vi "Hoff_cleaned.vi"(0 "Skip-1":i32=1, 2 "Image Pixels (U8)":u8[][](array[numeric])) -> (1 "3 times averaged":i32[][](graph), 5 "X Intercept":i32, 6 "Angle":i32, 7 "X Intercept 2":i32, 8 "Angle 2":i32)   [LabVIEW 2009]
panel:
  in  "Angle Canceling Resolution":i32=20
  in  "X Intercept Canceling Resolution":i32=200
  in  "Xintercept Pixel Resolution":dbl=20.0
  out "Vector Reformat":i32[][](array[numeric])
  out "Intensity Graph":i32[][](graph)
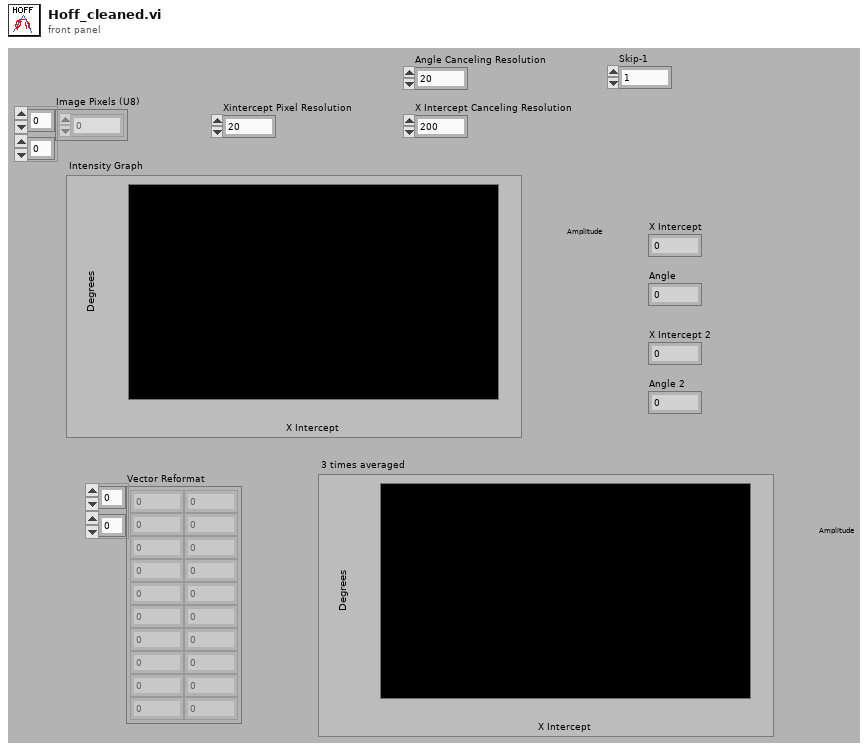
[diagram p1: front panel]
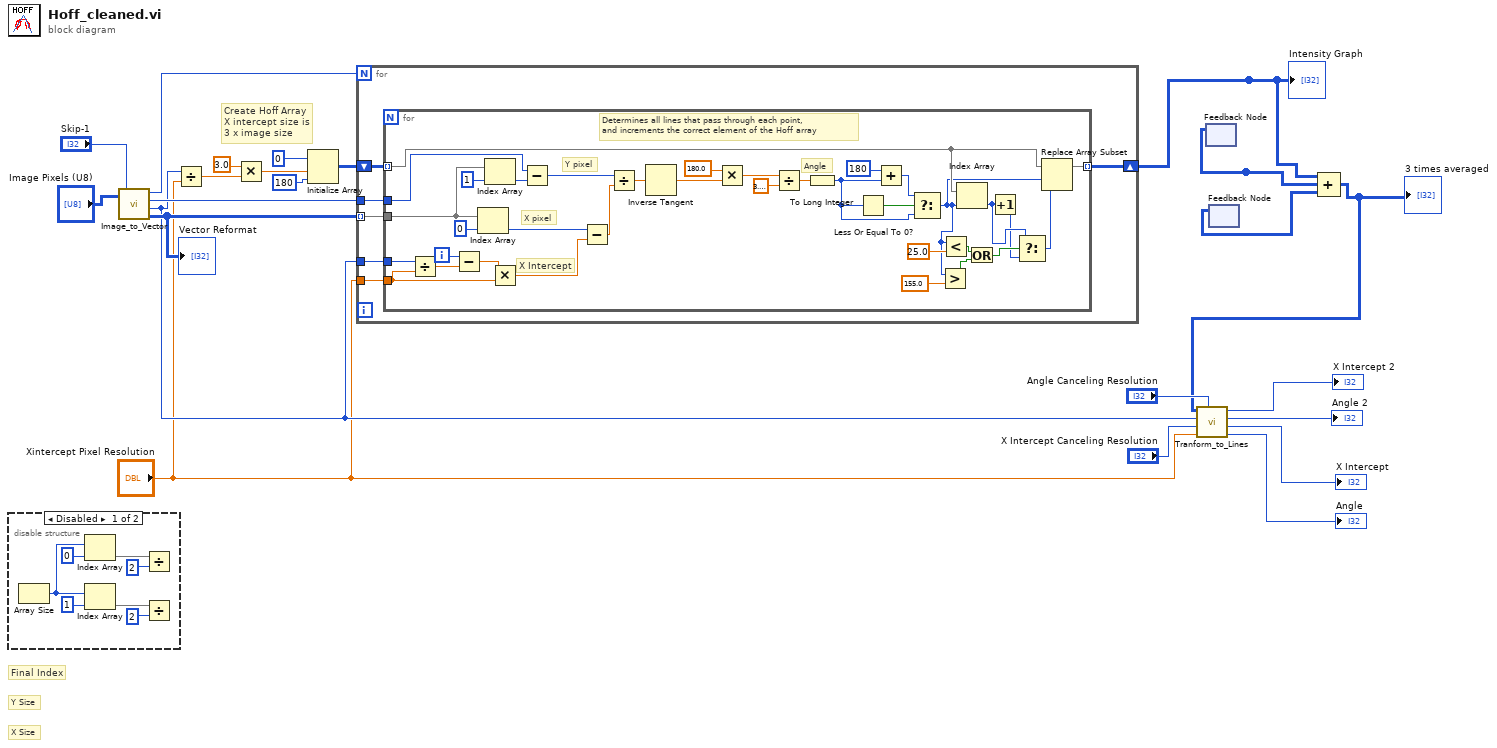
[diagram p0: block diagram]
diagram:
  # "Create Hoff Array\nX intercept size is \n3 x image size"
  # "Final Index"
  # "Y Size"
  # "X Size"
  n1 = disable-structure shown="Disabled" {
    frame #0 {
      n2 = Array Size() -> (size(s)=w32:i32)  [unwired: 1 in]
      n3 = Index Array(array=w32, index=0) -> (element=w29)
      n4 = Index Array(array=w32, index=1) -> (element=w26)
      n5 = Divide(x=w29, y=2) -> (x/y=w25:dbl)
      n6 = Divide(x=w26, y=2) -> (x/y=w24:dbl)
    }
    frame #1 {
    }
  }
  n7 = call "Image_to_Vector.vi"("Image Pixels (U8)"="Image Pixels (U8)", "Skip-1"="Skip-1") -> ("Final Index"=w18:i32, "Y Size"=w17:i32, "X Size"=w13:i32, "Vector Format"=w19:i32[][])
  "Vector Reformat" <- w19
  n8 = Divide(x=w13, y="Xintercept Pixel Resolution") -> (x/y=w16:dbl)
  n9 = Multiply(x=3.0 ("y"), y=w16) -> (x*y=w15:dbl)
  n10 = Initialize Array(0 ("element"), w15, 180 ("dimension size")) -> (w20:i32[][])
  n11 = for {
    N: w18 -> [_]
    tunnel: w13 -> [w37]
    tunnel: w19 -> [w36] mode=indexing
    tunnel: w17 -> [w35]
    shift-right: [w34] -> w5
    shift-left: w20 -> [w38]
    tunnel: "Xintercept Pixel Resolution" -> [w33]
    n12 = for {
      tunnel: w37 -> [w49]
      tunnel: w36 -> [w58]
      tunnel: w35 -> [w56]
      tunnel: w38 -> [w73] mode=indexing
      tunnel: [w53] -> w34 mode=indexing
      tunnel: w33 -> [w48]
      i -> [w66]
      # "Determines all lines that pass through each point,\nand increments the correct element of the Hoff array"
      # "X pixel"
      # "Y pixel"
      # "Angle"
      # "X Intercept"
      n13 = Divide(x=w49, y=w48) -> (x/y=w50:dbl)
      n14 = Subtract(x=w66, y=w50) -> (x-y=w52:dbl)
      n15 = Index Array(array=w58, index=0) -> (element=w57:i32)
      n16 = Index Array(array=w58, index=1) -> (element=w55:i32)
      n17 = Multiply(x=w52, y=w48) -> (x*y=w51:dbl)
      n18 = Subtract(x=w56, y=w55) -> (x-y=w54:i32)
      n19 = Subtract(x=w57, y=w51) -> (x-y=w72:dbl)
      n20 = Divide(x=w54, y=w72) -> (x/y=w68:dbl)
      n21 = Inverse Tangent(1:w68) -> (0:w67:dbl)
      n22 = Multiply(x=180.0 ("y"), y=w67) -> (x*y=w69:dbl)
      n23 = Divide(x=w69, y=3.141592653589793) -> (x/y=w70:dbl)
      n24 = To Long Integer(number=w70) -> (32bit integer=w62:i32)
      n25 = Less Or Equal To 0?(x=w62) -> (x <= 0?=w64:bool)
      n26 = Add(x=180, y=w62) -> (x+y=w61:i32)
      n27 = Select(t=w61, s=w64, f=w62) -> (s? t:f=w41:i32)
      n28 = Greater?(x=w41, y=155.0) -> (0:w46:bool)
      n29 = Less?(x=w41, y=25.0) -> (x < y?=w47:bool)
      n30 = Index Array(array=w73, index=w41) -> (element=w40:i32)
      n31 = Or(x=w47, y=w46) -> (x .or. y?=w45:bool)
      n32 = Increment(x=w40) -> (x+1=w39:i32)
      n33 = Select(t=w40, s=w45, f=w39) -> (s? t:f=w44:i32)
      n34 = Replace Array Subset(array=w73, new element=w44, index=w41) -> (w53:i32[])
    }
  }
  "Intensity Graph" <- w5
  n35 = feedback #1() -> (w4:i32[][])  [unwired: 1 out]
  n36 = feedback #2() -> (w3:i32[][])  [unwired: 1 out]
  n37 = Compound Arithmetic op=ADD(w5, w4, w3) -> (w2:i32[][])
  "3 times averaged" <- w2
  n38 = call "Tranform_to_Lines.vi"("Angle Canceling Resolution"="Angle Canceling Resolution", "Xintercept Pixel Resolution"="Xintercept Pixel Resolution", "X Intercept Canceling Resolution"="X Intercept Canceling Resolution", "X Size"=w13, "Transformed Array"=w2) -> ("Angle 1"=→"Angle":i32, "X Intercept 1"=→"X Intercept":i32, "Angle 2"=→"Angle 2":i32, "X Intercept 2"=→"X Intercept 2":i32)
